vi "AgNA_Channel Measurement Marker Query Value.vi"(8 "error in (no error)":errorcluster {"code" format="%.0x"}, 9 "RepCapIdentifier":string, 11 "instrument handle":refnum<k15>) -> (0 "error out":errorcluster {"code" format="%.0x"}, 1 "pImagVal":dbl, 2 "pRealVal":dbl, 3 "instrument handle out":refnum<k15>)   [LabVIEW 2015]
uses:
  <instrlib>/Agilent NA/Agilent NA.lvlib
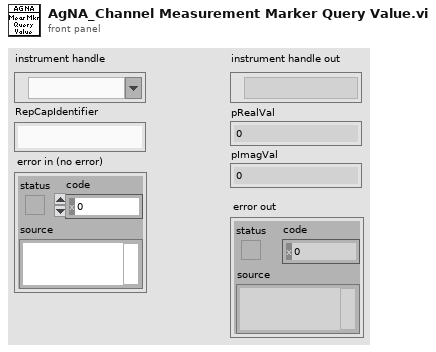
[diagram p1: front panel]
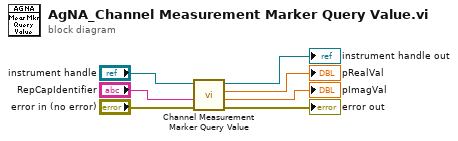
[diagram p0: block diagram]
diagram:
  n1 = call <instrlib>:"Channel Measurement Marker Query Value.vi"("error in (no error)"="error in (no error)", "RepCapIdentifier"="RepCapIdentifier", "instrument handle"="instrument handle") -> ("error out"=→"error out":errorcluster, "pImagVal"=→"pImagVal":dbl, "pRealVal"=→"pRealVal":dbl, "instrument handle out"=→"instrument handle out":refnum<k15>)  [unwired: 5 in]
